vi "DPO_7K_OpenVISA and Default Settings.vi"(8 "Error In":errorcluster, 11 "VISA resource name in":refnum<visa-resource-name>) -> (0 "error out":errorcluster, 3 "VISA resource name out":refnum<visa-resource-name>)   [LabVIEW 2020]
doc: "Establishes communication with the instrument and optionally performs an instrument identification query or an instrument reset. This VI also places the instrument in a default state needed for other instrument driver operations.\nRun this VI before running other instrument driver VIs for the instrument. You generally need to run the Initialize VI only once, at the beginning of an application."
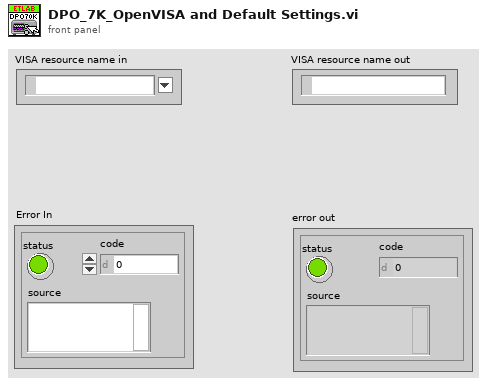
[diagram p1: front panel]
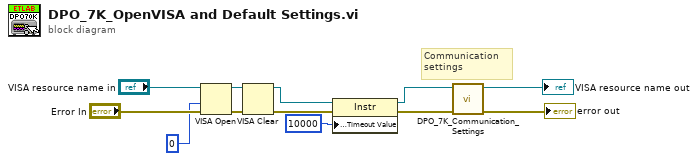
[diagram p0: block diagram]
diagram:
  # "Communication\nsettings"
  n1 = VISA Open(access mode=u32 0, error in (no error)="Error In", VISA resource name="VISA resource name in") -> (VISA resource name=w10:refnum<visa-resource-name>, error out=w9:errorcluster)  [unwired: 2 in]
  n2 = VISA Clear(VISA resource name=w10, error in (no error)=w9) -> (VISA resource name out=w8:refnum<visa-resource-name>, error out=w7:errorcluster)
  n3 = property on="Property Node" class="Instr"(reference=w8, error in=w7, "General Settings:Timeout Value"=u32 10000) -> (reference out=w3:refnum<visa-resource-name>, error out=w4:errorcluster)
  n4 = call "DPO_7K_Communication_Settings.vi"("Error In"=w4, "VISA resource name in"=w3) -> ("error out"=→"error out":errorcluster, "VISA resource name out"=→"VISA resource name out":refnum<visa-resource-name>)  [unwired: 8 in]
